vi "Emballage_BDD_adresseIPImprimante_NomImprimante.vi"(8 "Error in":errorcluster caption="Error in (no error)", 11 "ADRESSE_IP":string) -> (0 "Error out":errorcluster, 3 "NOM":string)   [LabVIEW 2020]
uses:
  Modules/FS/60_FS_Controles/60_FS_SetGet.ctl
  <vilib>/drjdpowell/SQLite Library/SQL Connection/Open (path).vi
  <vilib>/drjdpowell/SQLite Library/SQL Connection/Open (string).vi
  <vilib>/AdvancedString/Path To Command Line String.vi
  <vilib>/drjdpowell/SQLite Library/SQL Connection/Connection.lvclass
panel:
  out "Result Set":string[][](table) caption="Result Set (from first statement with results)"
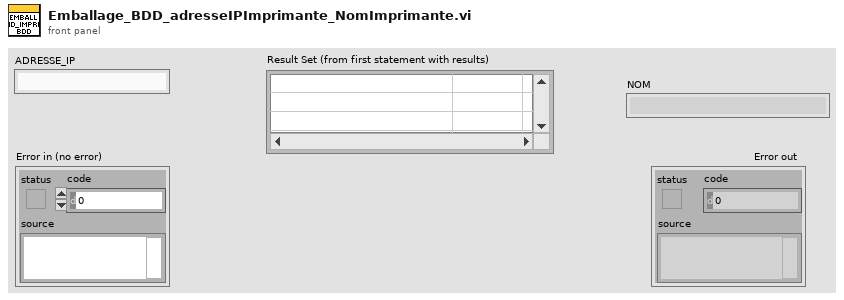
[diagram p1: front panel]
types:
  T1 = typedef "60_FS_SetGet.ctl" = enum16{"set", "get"}
  T2 = typedef "60_FS_CLT_Chemins.ctl" = cluster{"Racine_local":path, "Racine_reseau":path, "Racine_Support_Application":path, "Fichier_Journalisation":path, "Connexion_BDD_VSX":path, "Connexion_BDD_PLZ":path}
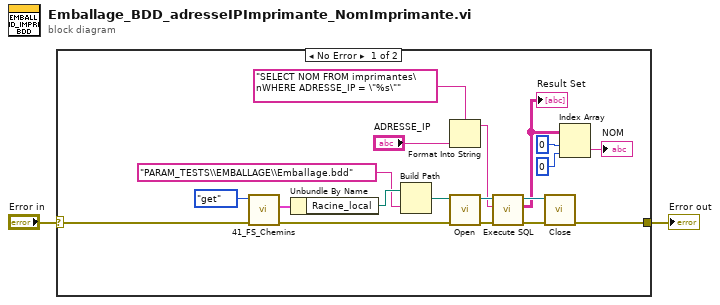
[diagram p0: block diagram]
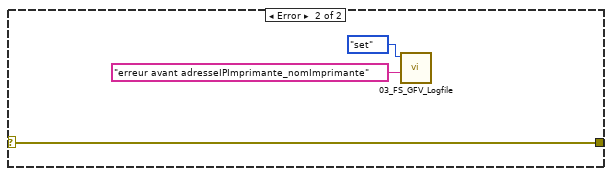
[diagram p2: hidden frame]
diagram:
  n1 = case shown="No Error" "Error in" {
    selector: "Error in" -> [w4 w24]
    tunnel: [w3 w24] -> w1
    frame No Error {
      n2 = call "41_FS_Chemins.vi"("error in (no error)"=w4, "SetGet"=60_FS_SetGet."get") -> ("error out"=w18:errorcluster, "CLT_Chemins_out"=w20:T2)  [unwired: 8 in]
      n3 = Unbundle By Name(w20) -> ("Racine_local"=w19:path)
      n4 = Build Path(base path=w19, name or relative path="PARAM_TESTS\\EMBALLAGE\\Emballage.bdd" ("nom ou chemin relatif")) -> (appended path=w10:path)
      n5 = Format Into String(format string="SELECT NOM FROM imprimantes\nWHERE ADRESSE_IP = \"%s\"" ("SQL"), "ADRESSE_IP") -> (resulting string=w11:string)  [unwired: 2 in, 1 out]
      n6 = call-poly <vilib>:"Open.vi"("error in (no error)"=w18, "db file"=w10) -> ("error out"=w17:errorcluster, "SQLite Connection"=w16:refnum<class "Connection.lvclass">)  [unwired: 8 in]
      n7 = call <vilib>:"Execute SQL.vi"("error in (no error)"=w17, "SQL"=w11, "SQLite Connection in"=w16) -> ("error out"=w15:errorcluster, "Result Set"=w8:string[][], "SQLite Connection"=w14:refnum<class "Connection.lvclass">)  [unwired: 5 in, 1 out]
      "Result Set" <- w8
      n8 = call-dynamic "Close.vi"("error in (no error)"=w15, "SQLite Connection in"=w14) -> ("error out"=w3:errorcluster)  [unwired: 9 in]
      n9 = Index Array(array=w8, index (row)=0 ("indice (ligne)"), index (col)=0 ("indice désactivé (col)")) -> (element=→"NOM":string)
    }
    frame Error {
      n10 = call "03_FS_GFV_Logfile.vi"("Chaîne"="erreur avant adresseIPImprimante_nomImprimante", "States"=60_FS_SetGet."set") -> ()  [unwired: 8 in, 2 out]
    }
  }
  "Error out" <- w1
